vi "startWorld.vi"(6 "axisLength":dbl=150.0, 11 "SceneObjectIn":refnum<vi>) -> (0 "error out":errorcluster, 2 "axesOut":refnum<vi>, 3 "SceneObject out":refnum<vi>)   [LabVIEW 2022 SP3]
uses:
  <vilib>/picture/3D Picture Control/Object/Create Object (name).vi
  <vilib>/picture/3D Picture Control/NI_3D Picture Control.lvlib
  <vilib>/picture/3D Picture Control/Object/Add Object (reference).vi
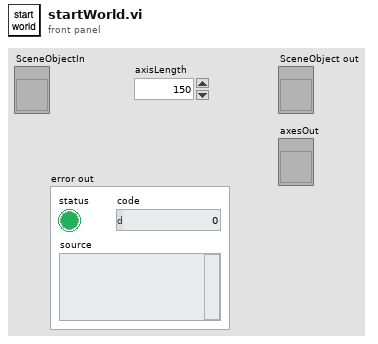
[diagram p1: front panel]
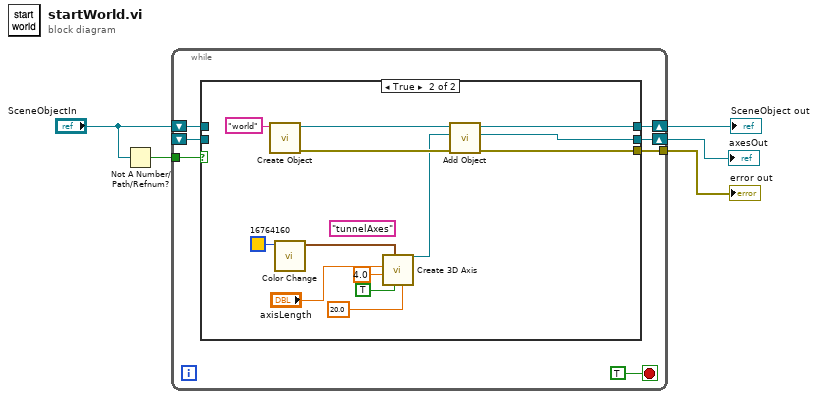
[diagram p0: block diagram]
diagram:
  n1 = Not A Number/Path/Refnum?(number/path/refnum="SceneObjectIn") -> (NaN/Path/Refnum?=w3:bool)
  n2 = while {
    tunnel: [w12] -> w5
    tunnel: w3 -> [w10]
    shift-right: [w11] -> w4
    shift-left: "SceneObjectIn" -> [w9]
    shift-right: [w8] -> w1
    shift-left: _ -> [w7]
    stop <- TRUE stop-if-true
    n3 = case shown="True" w10 {
      tunnel: [_ w15] -> w12
      tunnel: [w14 w16] -> w11
      tunnel: w9 -> [w14 _]
      tunnel: [w13 w17] -> w8
      tunnel: w7 -> [w13 _]
      frame False {
      }
      frame True {
        (unwired) "tunnelAxes" ("Name")
        n4 = call-poly <vilib>:"Create Object.vi"("Name"="world") -> ("error out"=w19:errorcluster, "Scene:New Object"=w20:refnum<vi>)  [unwired: 9 in]
        n5 = call <vilib>:"Color Change.vi"("Color"=u32 16764160) -> ("RGBA"=w23:cluster{"R":sgl, "G":sgl, "B":sgl, "A":sgl})  [unwired: 10 in]
        n6 = call <vilib>:"Create 3D Axis.vi"("Character Size"=sgl 20.0, "Axis label?"=TRUE, "Color"=w23, "Radius"=sgl 4.0, "Length"="axisLength") -> ("New Object Refnum"=w18:refnum<vi>)  [unwired: 5 in, 1 out]
        n7 = call-poly <vilib>:"Add Object.vi"("error in (no error)"=w19, "New Object In"=w18, "Scene Object In"=w20) -> ("error out"=w15:errorcluster, "New Object Out"=w17:refnum<vi>, "Scene Object Out"=w16:refnum<vi>)  [unwired: 6 in]
      }
    }
  }
  "error out" <- w5
  "SceneObject out" <- w4
  "axesOut" <- w1
